vi "set_scan_specification.vi"(8 "error in (no error)":errorcluster, 10 "scan specification":T1, 11 "FPGA_AK101022Resonance in":refnum<class "FPGAWrapperAK101022Resonance.lvclass">) -> (0 "error out":errorcluster, 3 "FPGA_AK101022Resonance out":refnum<class "FPGAWrapperAK101022Resonance.lvclass">)   [LabVIEW 2010, in "FPGAWrapperAK101022Resonance.lvclass"]
uses:
  FPGAWrapperAK101022Resonance.lvclass
  scan_specification_cluster.ctl
  class_data.vi
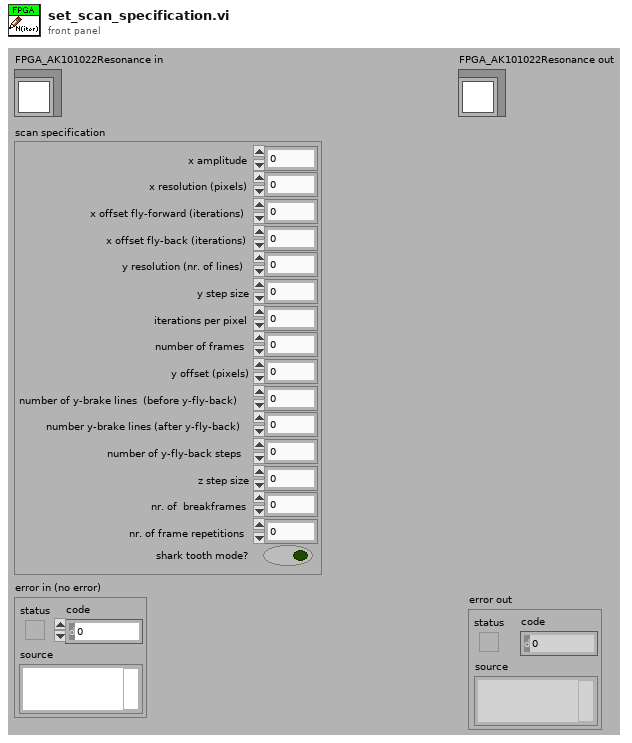
[diagram p1: front panel]
types:
  T1 = typedef "scan_specification_cluster.ctl" = cluster{"x amplitude":u16, "x resolution (pixels)":u16, "x offset fly-forward (iterations)":u16, "x offset fly-back (iterations)":u16, "y resolution (nr. of lines)":u16, "y step size":u16, "iterations per pixel":u16, "number of frames":i32, "y offset (pixels)":u16, "number of y-brake lines  (before y-fly-back)":u16, "number y-brake lines (after y-fly-back)":u16, "number of y-fly-back steps":u16, "z step size":u16, "nr. of  breakframes":u16, "nr. of frame repetitions":u16, "shark tooth mode?":bool}
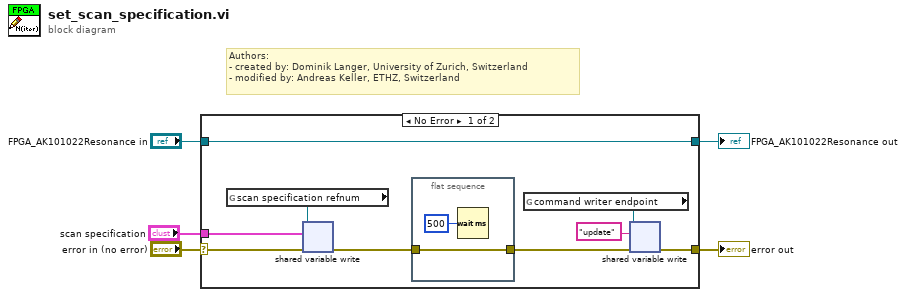
[diagram p0: block diagram]
diagram:
  # "Authors: \n- created by: Dominik Langer, University of Zurich, Switzerland\n- modified by: Andreas Keller, ETHZ, Switzerland"
  n1 = case shown="No Error" "error in (no error)" {
    selector: "error in (no error)" -> [w8 w18]
    tunnel: [w13 w18] -> w3
    tunnel: [w14 w17] -> w2
    tunnel: "FPGA_AK101022Resonance in" -> [w14 w17]
    tunnel: "scan specification" -> [w6 _]
    frame No Error {
      n2 = global read "class_data.vi" "scan specification refnum"() -> (w9:refnum<k21>)
      n3 = shared-variable-write(w9, w8, w6) -> (w7:errorcluster)  [unwired: 1 out]
      n4 = flat-sequence {
        tunnel: w7 -> [w15]
        tunnel: [w15] -> w10
        frame #0 {
          n5 = Wait (ms)(milliseconds to wait=u32 500) -> ()  [unwired: 1 out]
        }
      }
      n6 = global read "class_data.vi" "command writer endpoint"() -> (w12:refnum<k21>)
      n7 = shared-variable-write(w12, w10, "update" ("data in")) -> (w13:errorcluster)  [unwired: 1 in, 2 out]
    }
    frame Error {
    }
  }
  "error out" <- w3
  "FPGA_AK101022Resonance out" <- w2
